vi "Generate New Parameter Fit.vi"(6 "Rearranged Parameter Fit":dbl[][](array[numeric]), 7 "Status":i32[](array[numeric]), 8 "List ROI In":dbl[][](array[numeric])=[[2.29530433588858, 0.13476419761712136, 745.0, 787.0, 2.2274995965883164, 2.3624656364482517, 7971.631104776367, 629.6678820155158], [3.6923878537448513, 0.1335886705835358, 1180.0, 1222.0, 3.625362152280503, 3.760328192140438, 67874.85518278569, 664.4170311995598], [4.0147539339226315, 0.13386763074225186, 1280.0, 1322.0, 3.9467098662327302, 4.0816759060926655, 9216.928010954993, 599.404820008226]], 9 "List MultiFit In":dbl[][](array[numeric]), 10 "All FWHM":dbl[](array[numeric]), 11 "All Parameters Fit":T1(array[cluster])) -> (0 "List ROI Out":dbl[][](array[numeric]), 1 "List MultiFit Out":dbl[][](array[numeric]))   [LabVIEW 2023]
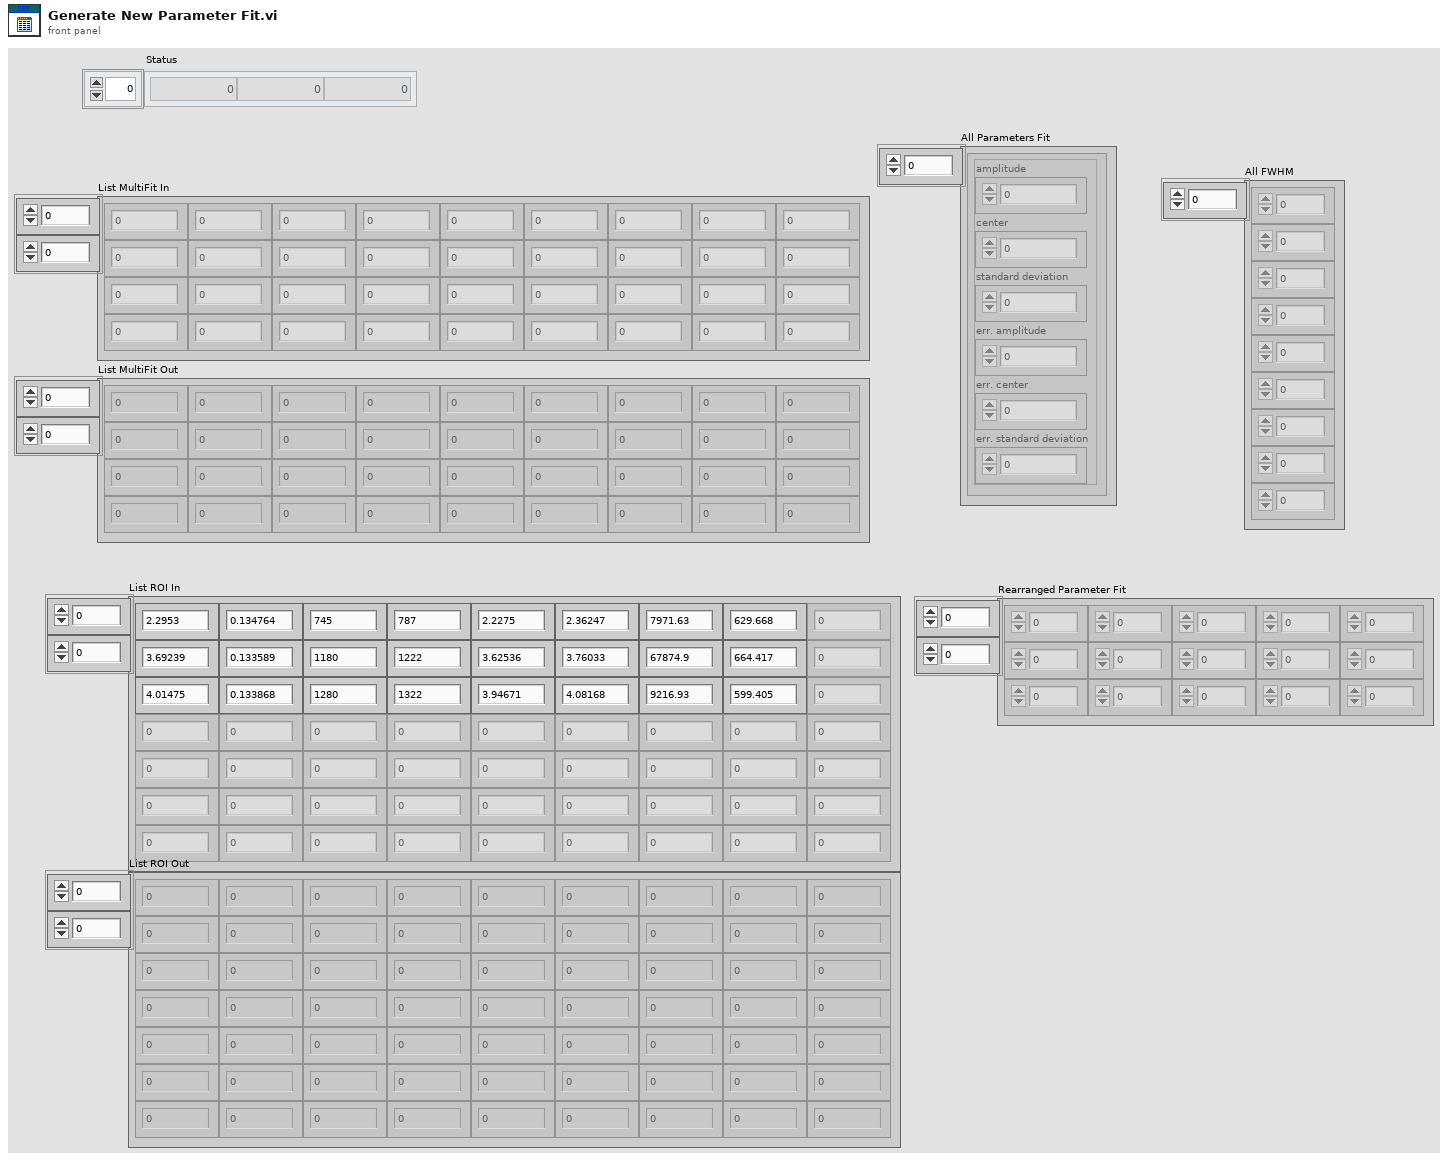
[diagram p1: front panel]
types:
  T1 = cluster{"amplitude":dbl, "center":dbl, "standard deviation":dbl, "err. amplitude":dbl, "err. center":dbl, "err. standard deviation":dbl}[]
  T2 = cluster{"amplitude":dbl, "center":dbl, "standard deviation":dbl, "offset":dbl, "err. amplitude":dbl, "err. center":dbl, "err. standard deviation":dbl, "err. offset":dbl}
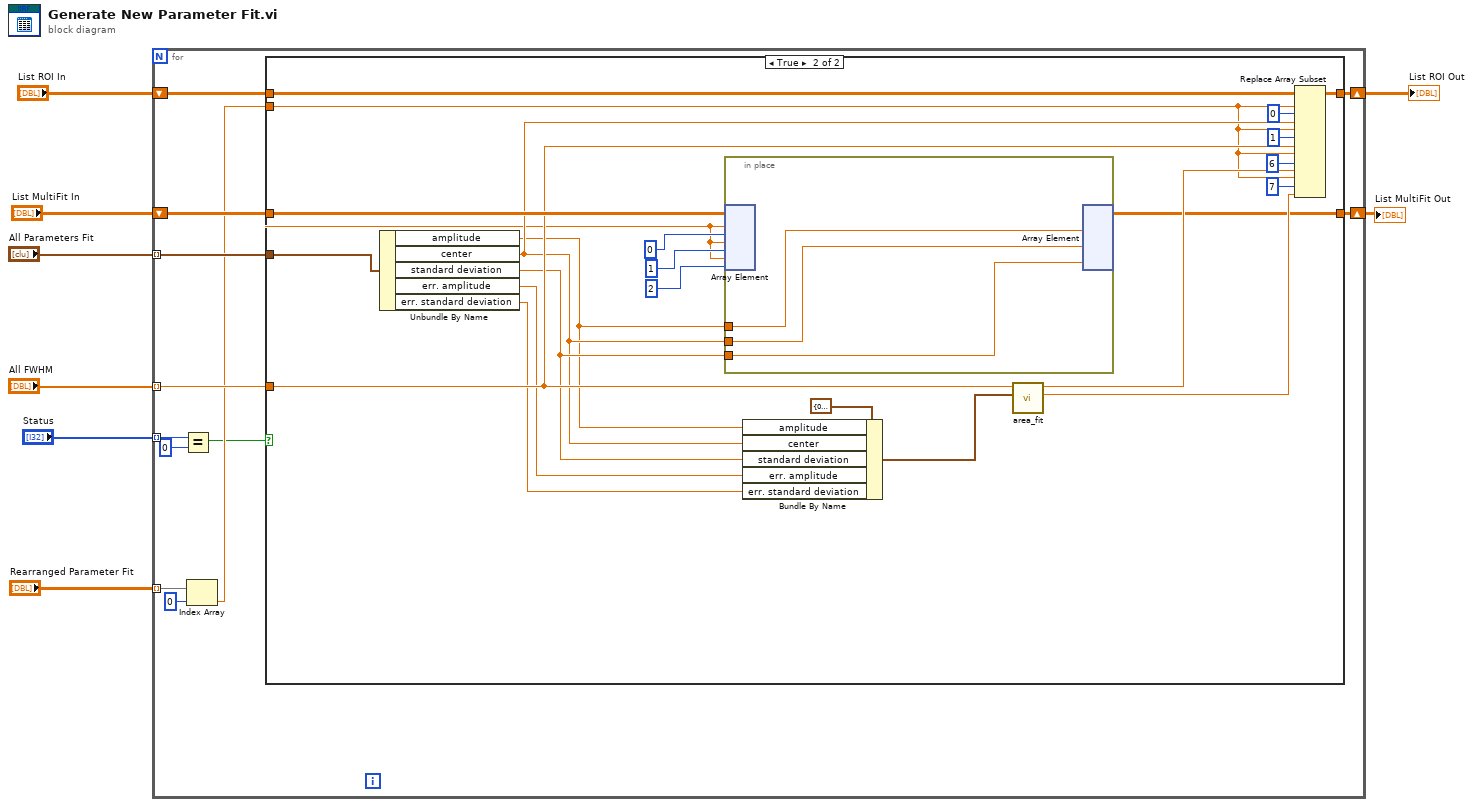
[diagram p0: block diagram]
diagram:
  n1 = for {
    tunnel: "All Parameters Fit" -> [w20] mode=indexing
    tunnel: "All FWHM" -> [w17] mode=indexing
    tunnel: "Rearranged Parameter Fit" -> [w16] mode=indexing
    shift-right: [w18] -> w4
    shift-left: "List ROI In" -> [w14]
    shift-right: [w12] -> w2
    shift-left: "List MultiFit In" -> [w19]
    tunnel: "Status" -> [w11] mode=indexing
    n2 = Equal?(x=w11, y=0) -> (x = y?=w9:bool)
    n3 = Index Array(array=w16, index=0) -> (element=w13:dbl)
    n4 = case shown="True" w9 {
      tunnel: w20 -> [_ w45]
      tunnel: w19 -> [w21 w44]
      tunnel: [w22 w43] -> w18
      tunnel: w17 -> [_ w40]
      tunnel: w14 -> [w22 w28]
      tunnel: w13 -> [_ w24]
      tunnel: [w21 w23] -> w12
      frame False {
      }
      frame True {
        n5 = Unbundle By Name(w45) -> ("amplitude"=w33:dbl, "center"=w34:dbl, "standard deviation"=w35:dbl, "err. amplitude"=w37:dbl, "err. standard deviation"=w36:dbl)
        n6 = in-place {
          in-place-border: w33 -> [w48]
          in-place-border: w34 -> [w47]
          in-place-border: w35 -> [w46]
          n7 = in-place-array #1(w44, w24, 0, w24, 1, w24, 2) -> ()  [unwired: 3 out]
          n8 = in-place-array #1(w48, w47, w46) -> (w23:dbl[][])  [unwired: 6 out]
        }
        n9 = Bundle By Name(cluster=T2 {"amplitude"=0.0, "center"=0.0, "standard deviation"=0.0, "offset"=0.0, "err. amplitude"=0.0, "err. center"=0.0, "err. standard deviation"=0.0, "err. offset"=0.0} ("Parameters Fit"), "amplitude"=w33, "center"=w34, "standard deviation"=w35, "err. amplitude"=w37, "err. standard deviation"=w36) -> (w38:T2)
        n10 = call "area_fit.vi"("Parameters Fit"=w38, "FWHM"=w40) -> ("Err. Area"=w29:dbl, "Area"=w30:dbl)  [unwired: 8 in]
        n11 = Replace Array Subset(array=w28, new element #1=w34, index (row) #1=w24, index (col) #1=0 ("index"), new element #2=w40, index (row) #2=w24, index (col) #2=1 ("index"), new element #3=w30, index (row) #3=w24, index (col) #3=6 ("index"), new element #4=w29, index (row) #4=w24, index (col) #4=7 ("index")) -> (w43:dbl[][])
      }
    }
  }
  "List ROI Out" <- w4
  "List MultiFit Out" <- w2
